vi "justOneBlank.vi"(1 "TF":bool=TRUE, 2 "input":string) -> (0 "output":string)   [LabVIEW 2011]
panel:
  out "flag_1":i32
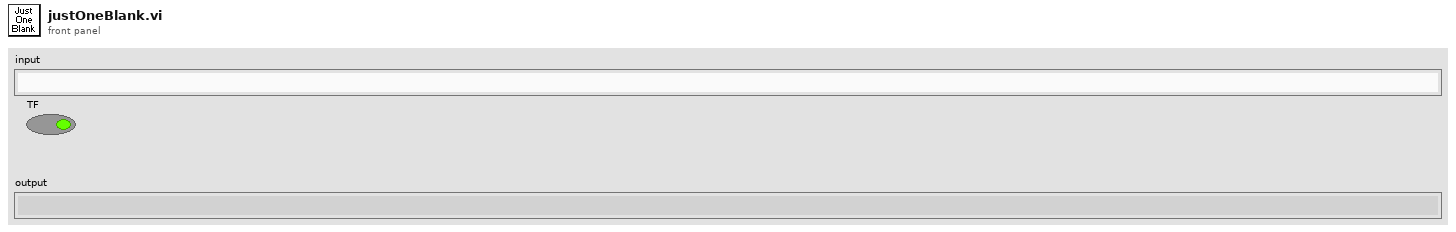
[diagram p1: front panel]
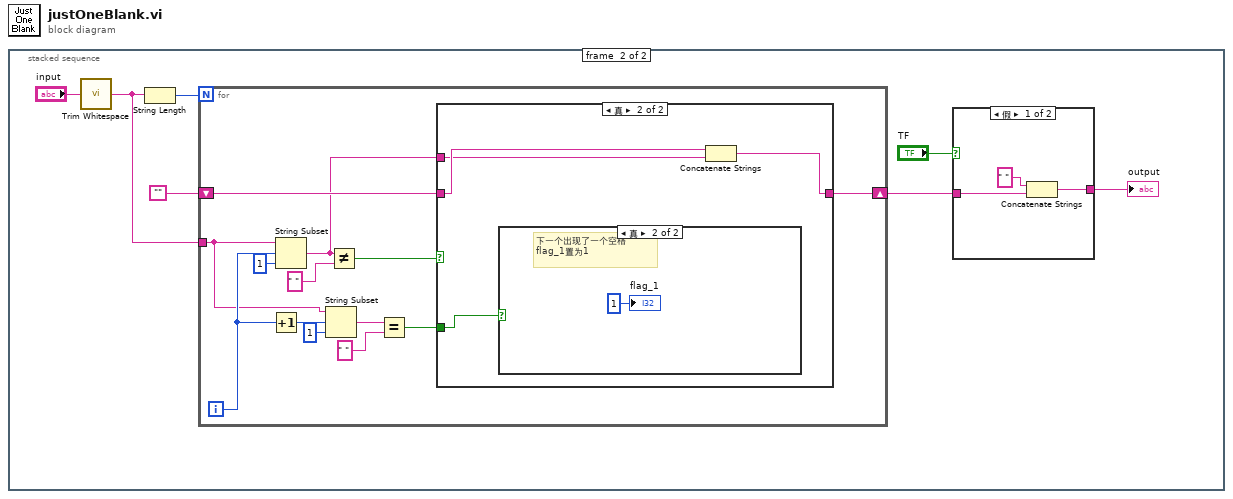
[diagram p0: block diagram]
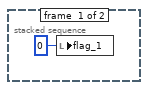
[diagram p2: hidden frame]
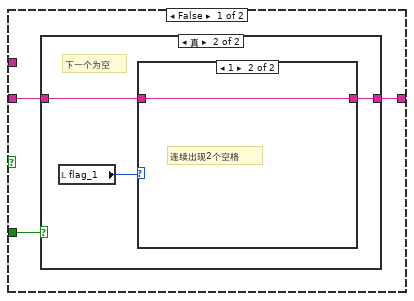
[diagram p4: hidden frame]
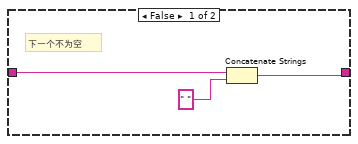
[diagram p5: hidden frame]
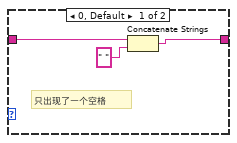
[diagram p6: hidden frame]
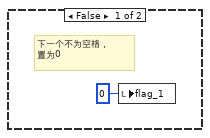
[diagram p7: hidden frame]
diagram:
  n1 = stacked-sequence {
    frame #0 {
      n2 = local write "flag_1"(0 ("flag_1")) -> ()
    }
    frame #1 {
      n3 = call <vilib>:"Trim Whitespace.vi"("string"="input") -> ("trimmed string"=w6:string)  [unwired: 1 in]
      n4 = String Length(string=w6) -> (length=w8:i32)
      n5 = for {
        N: w8 -> [_]
        tunnel: w6 -> [w13]
        shift-right: [w15] -> w4
        shift-left: "" -> [w16]
        i -> [w22]
        n6 = Increment(x=w22) -> (x+1=w18:i32)
        n7 = String Subset(string=w13, offset (0)=w22, length (rest)=1 ("长度（剩余）")) -> (substring=w14:string)
        n8 = String Subset(string=w13, offset (0)=w18, length (rest)=1 ("长度（剩余）")) -> (substring=w20:string)
        n9 = Not Equal?(x=w14, y=" ") -> (x != y?=w23:bool)
        n10 = Equal?(x=w20, y=" ") -> (x = y?=w17:bool)
        n11 = case shown="真" w23 {
          tunnel: w17 -> [w28 w42]
          tunnel: w16 -> [w27 w40]
          tunnel: [w26 w41] -> w15
          tunnel: w14 -> [_ w39]
          frame False {
            n12 = case shown="真" w28 {
              tunnel: w27 -> [w31 w33]
              tunnel: [w30 w32] -> w26
              frame False {
                # "下一个不为空"
                n13 = Concatenate Strings(w31, " " ("字符串")) -> (w30:string)
              }
              frame True {
                # "下一个为空"
                n14 = local read "flag_1"() -> (w34:i32)
                n15 = case shown="1" w34 {
                  tunnel: w33 -> [w37 w38]
                  tunnel: [w36 w38] -> w32
                  frame 0, Default {
                    # "只出现了一个空格"
                    n16 = Concatenate Strings(w37, " " ("字符串")) -> (w36:string)
                  }
                  frame 1 {
                    # "连续出现2个空格"
                  }
                }
              }
            }
          }
          frame True {
            n17 = case shown="真" w42 {
              frame False {
                # "下一个不为空格，\n置为0"
                n18 = local write "flag_1"(0 ("flag_1")) -> ()
              }
              frame True {
                # "下一个出现了一个空格\nflag_1置为1"
                "flag_1" <- 1 ("flag")
              }
            }
            n19 = Concatenate Strings(w40, w39) -> (w41:string)
          }
        }
      }
      n20 = case shown="假" "TF" {
        tunnel: w4 -> [w11 w12]
        tunnel: [w10 w12] -> w3
        frame False {
          n21 = Concatenate Strings(" " ("字符串"), w11) -> (w10:string)
        }
        frame True {
        }
      }
      "output" <- w3
    }
  }
